vi "Execute.LoadSequences.vi"(8 "error in (no error)":errorcluster, 11 "Cluster":T1={"NIVS.BaseLogPath"=path "", "NIVS.SystemDefinitionFile"=path "", "NIVS.Events"={"SequenceEvent"=refnum, "SystemChangeEvent"=refnum, "WorkspaceEvent"=refnum}, "NIVS.SequenceState"=enum."Idle", "NIVS.GatewayIPAddress"="", "NIVS.DataLogSpecRef"=refnum, "NIVS.DataLogManagerRef"=refnum, "NIVS.LogSessionGUID"="", "NIVS.WorkspaceManager"=refnum, "NIVS.Deployed"=FALSE, "NIVS.ProfileRef"=refnum, "NIVS.ProfileCallback"=refnum, "NIVS.SystemStateRefs"={"CustDatRef"=refnum, "EvtRef"=refnum}, "UI.Abort"=refnum, "UI.Pause"=refnum, "UI.EnableLogging"=refnum, "UI.Start"=refnum, "UI.LogChannels"=refnum, "UI.StartIteration"=refnum, "UI.StartStep"=refnum, "UI.Sequence"=refnum, "UI.PreviewMode"=refnum, "UI.Graph"=refnum, "UI.BaseFileName"=refnum, "UI.Profiles"=refnum, "UI.CurrentStep"=refnum, "UI.CurrentIteration"=refnum, "UI.TotalIterations"=refnum, "Sequence.AbortChannel"="", "Sequence.StepInfoChannel"="", "Sequence.Iterations"=0, "Sequence.IterationInfoChannel"="", "Sequence.#ofColumns"=0, "Events.State"=refnum, "Events.Test Result"=refnum, "Events.Progress"=refnum, "INI.Settings"={"Build Location"=path "C:/Simple Sequence Editor/SequenceRepo", "LoggingLocation"=path ""}, "UI.Skip"=refnum, "Sequence.SkipChannel"="", "Restart.Path"=path "", "UI.Duration"=refnum, "Sequence.DurationChannel"=""}) -> (0 "error out":errorcluster)   [LabVIEW 2013, in "Simple Sequence Tools - Execution.lvlib"]
uses:
  Simple Sequence Tools - Execution.lvlib
  Types/Main.StateVariables.ctl
  Types/Execute.UserEventRefs.ctl
  <vilib>/NI Veristand/Execution/Workspace/SystemStateRegEventRef.ctl
  Types/Execution.SequenceState.ctl
  <vilib>/NI Veristand/Execution/DataLogging/DataLoggingSpecification Ref.ctl
  NationalInstruments.VeriStand.ClientAPI
  <vilib>/NI Veristand/Execution/DataLogging/IDataLogging Ref.ctl
  <vilib>/NI Veristand/Execution/Workspace/WorkspaceAPI.ctl
  NationalInstruments.VeriStand.RealTimeSequenceDefinitionApi
  <vilib>/NI Veristand/Execution/Workspace/SystemStateEventRef.ctl
  Shared/Types/INI.Settings
  Shared/Simple Sequence Tools - Shared.lvlib
  <vilib>/NI Veristand/Execution/Workspace/NI_VS Workspace ExecutionAPI.lvlib
  <vilib>/NI Veristand/Execution/DataLogging/NI_VS Data Logging API.lvlib
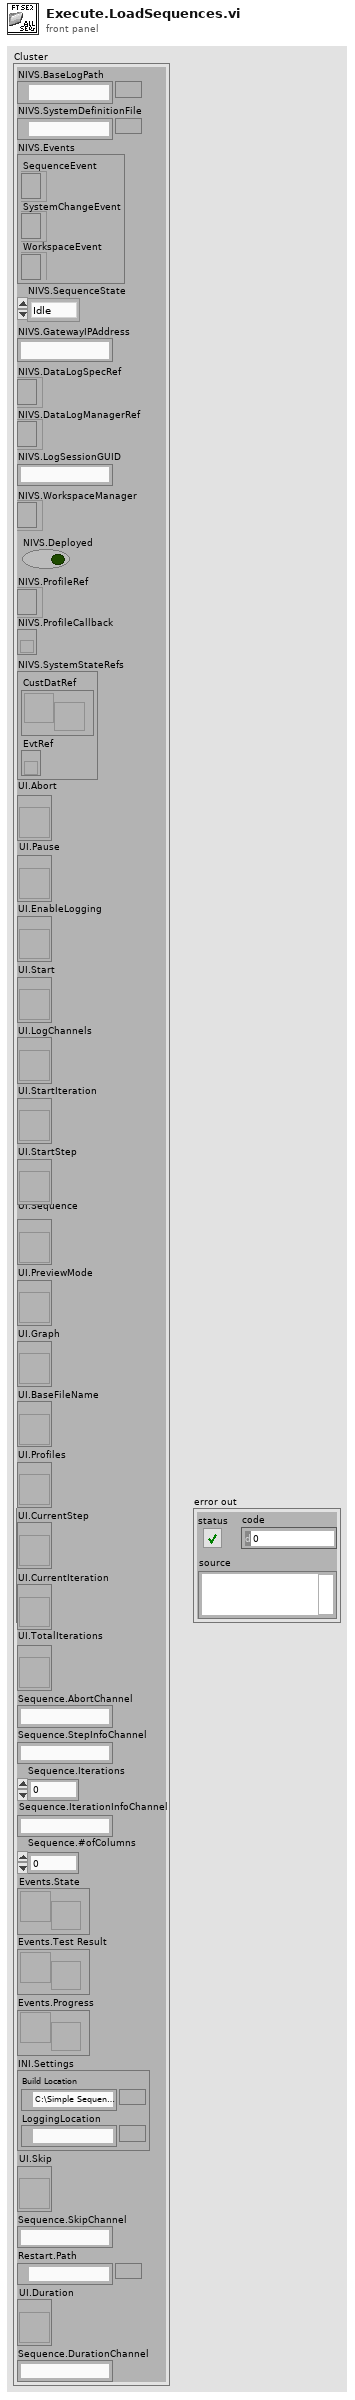
[diagram p1: front panel]
types:
  T1 = typedef "Simple Sequence Tools - Execution.lvlib/Main.StateVariables.ctl" = cluster{"NIVS.BaseLogPath":path, "NIVS.SystemDefinitionFile":path, "NIVS.Events":T2, "NIVS.SequenceState":T4, "NIVS.GatewayIPAddress":string, "NIVS.DataLogSpecRef":T5, "NIVS.DataLogManagerRef":T6, "NIVS.LogSessionGUID":string, "NIVS.WorkspaceManager":T7, "NIVS.Deployed":bool, "NIVS.ProfileRef":refnum<k24>, "NIVS.ProfileCallback":refnum<k27>, "NIVS.SystemStateRefs":T8, "UI.Abort":refnum<vi>, "UI.Pause":refnum<vi>, "UI.EnableLogging":refnum<vi>, "UI.Start":refnum<vi>, "UI.LogChannels":refnum<vi>, "UI.StartIteration":refnum<vi>, "UI.StartStep":refnum<vi>, "UI.Sequence":refnum<vi>, "UI.PreviewMode":refnum<vi>, "UI.Graph":refnum<vi>, "UI.BaseFileName":refnum<vi>, "UI.Profiles":refnum<vi>, "UI.CurrentStep":refnum<vi>, "UI.CurrentIteration":refnum<vi>, "UI.TotalIterations":refnum<vi>, "Sequence.AbortChannel":string, "Sequence.StepInfoChannel":string, "Sequence.Iterations":u32, "Sequence.IterationInfoChannel":string, "Sequence.#ofColumns":i32, "Events.State":refnum<user-event>, "Events.Test Result":refnum<user-event>, "Events.Progress":refnum<user-event>, "INI.Settings":T9, "UI.Skip":refnum<vi>, "Sequence.SkipChannel":string, "Restart.Path":path, "UI.Duration":refnum<vi>, "Sequence.DurationChannel":string}
  T2 = typedef "Simple Sequence Tools - Execution.lvlib/Execute.UserEventRefs.ctl" = cluster{"SequenceEvent":refnum<event-registration>, "SystemChangeEvent":T3, "WorkspaceEvent":refnum<event-registration>}
  T3 = typedef "NI_VS Workspace ExecutionAPI.lvlib/SystemStateRegEventRef.ctl" = refnum<event-registration>
  T4 = typedef "Simple Sequence Tools - Execution.lvlib/Execution.SequenceState.ctl" = enum16{"Idle", "Initializing", "Running", "Paused", "Finalizing", "Complete"}
  T5 = typedef "NI_VS Data Logging API.lvlib/DataLoggingSpecification Ref.ctl" = refnum<k24>
  T6 = typedef "NI_VS Data Logging API.lvlib/IDataLogging Ref.ctl" = refnum<k24>
  T7 = typedef "NI_VS Workspace ExecutionAPI.lvlib/WorkspaceAPI.ctl" = refnum<k24>
  T8 = typedef "NI_VS Workspace ExecutionAPI.lvlib/SystemStateEventRef.ctl" = cluster{"CustDatRef":refnum<user-event>, "EvtRef":refnum<k27>}
  T9 = typedef "Simple Sequence Tools - Shared.lvlib/INI.Settings" = cluster{"Build Location":path, "LoggingLocation":path}
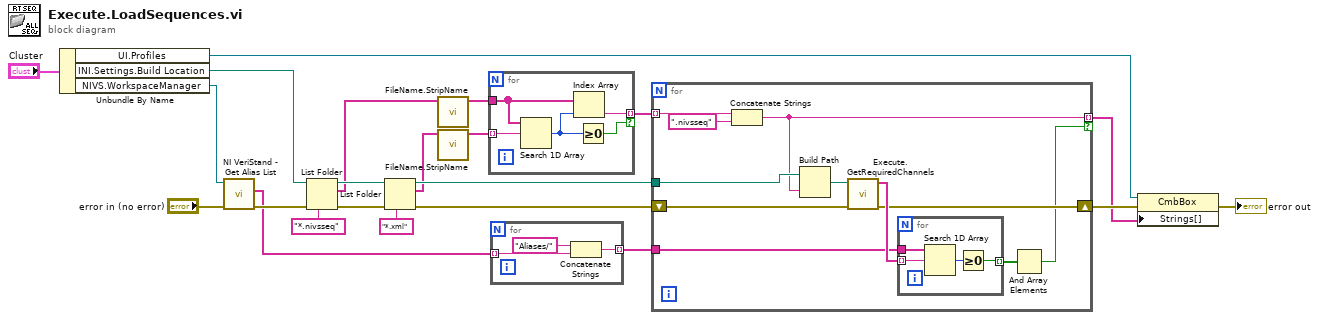
[diagram p0: block diagram]
diagram:
  n1 = Unbundle By Name("Cluster") -> ("UI.Profiles"=w20:refnum<vi>, "INI.Settings.Build Location"=w4:path, "NIVS.WorkspaceManager"=w17:T7)
  n2 = call <vilib>:"NI VeriStand - Get Alias List.vi"("error in (no error)"="error in (no error)", "WorkspaceManager in"=w17) -> ("error out"=w3:errorcluster, "Aliases"=w2:string[])  [unwired: 6 in, 2 out]
  n3 = List Folder(path=w4, pattern="*.nivsseq", error in=w3) -> (path out=w8:path, filenames=w6:string[], error out=w14:errorcluster)  [unwired: 1 in, 1 out]
  n4 = List Folder(path=w8, pattern="*.xml", error in=w14) -> (path out=w15:path, filenames=w7:string[], error out=w16:errorcluster)  [unwired: 1 in, 1 out]
  n5 = call "FileName.StripName.vi"("filenames"=w6) -> ("File name (no extension)"=w12:string[])  [unwired: 10 in]
  n6 = call "FileName.StripName.vi"("filenames"=w7) -> ("File name (no extension)"=w11:string[])  [unwired: 10 in]
  n7 = for {
    tunnel: w11 -> [w27] mode=indexing
    tunnel: w12 -> [w26]
    tunnel: [w24] -> w13 mode=indexing if=w23
    n8 = Search 1D Array(1D array=w26, element=w27) -> (index of element=w25:i32)  [unwired: 1 in]
    n9 = Index Array(array=w26, index=w25) -> (element=w24:string)
    n10 = Greater Or Equal To 0?(x=w25) -> (x >= 0?=w23:bool)
  }
  n11 = for {
    tunnel: w2 -> [w30] mode=indexing
    tunnel: [w28] -> w1 mode=indexing
    n12 = Concatenate Strings("Aliases/", w30) -> (w28:string)
  }
  n13 = for {
    tunnel: w13 -> [w41] mode=indexing
    tunnel: w15 -> [w39]
    shift-right: [w33] -> w19
    shift-left: w16 -> [w38]
    tunnel: w1 -> [w35]
    tunnel: [w32] -> w5 mode=indexing if=w31
    n14 = Concatenate Strings(w41, ".nivsseq" ("pattern")) -> (w32:string)
    n15 = Build Path(base path=w39, name or relative path=w32) -> (appended path=w37:path)
    n16 = call "Execute.GetRequiredChannels.vi"("error in (no error)"=w38, "Path"=w37) -> ("error out"=w33:errorcluster, "Channels"=w36:string[])  [unwired: 8 in]
    n17 = for {
      tunnel: w36 -> [w43] mode=indexing
      tunnel: w35 -> [w42]
      tunnel: [w44] -> w34 mode=indexing
      n18 = Search 1D Array(1D array=w42, element=w43) -> (index of element=w45:i32)  [unwired: 1 in]
      n19 = Greater Or Equal To 0?(x=w45) -> (x >= 0?=w44:bool)
    }
    n20 = And Array Elements(Boolean array=w34) -> (logical AND=w31:bool)
  }
  n21 = property class="CmbBox"(reference=w20, error in=w19, "Strings[]"=w5) -> (error out=→"error out":errorcluster)  [unwired: 1 out]
